vi "XML Script - Set Description of Existing Wire.vi"(9 "Description to Set":string, 10 "Wire Source":string, 11 "Code to Search":string) -> (2 "Wire found?":bool, 3 "Updated Code":string)   [LabVIEW 2017]
uses:
  <vilib>/_script/XML Scripting/XML Script Tag.ctl
  <vilib>/_script/XML Scripting/XML Script Attribute.ctl
panel:
  # "Set description on the first wire in \"Code to Search\"\nwhose source is Wire Source."
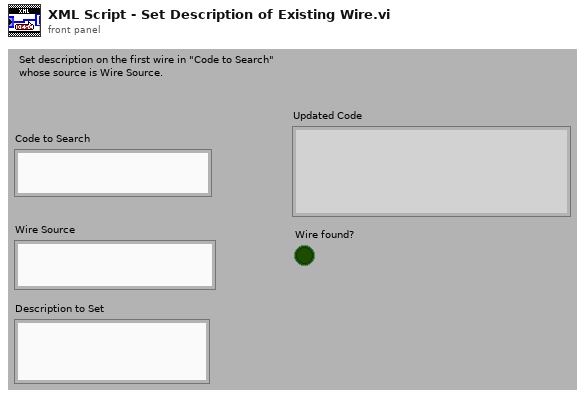
[diagram p1: front panel]
types:
  T1 = typedef "XML Script Attribute.ctl" = enum16{"name", "style", "path", "position", "in", "out", "width", "height", "index", "value", "default", "location", "offset", "typeindex", "size", "source", "destination", "indicator", "type", "controlname", "label", "conpaneidx", "mode", "description", "hasCondTerm", "linkIdentity", "caseselectortype", "concatInputs", "inName", "instantiationpath", "loopCondition", "IndexMode", "formulaInputs", "formulaOutputs", "msnFuncName", "msnIsDynamic", "msnIsODEUserFunction", "ignoreSearchDialog"}
  T2 = typedef "XML Script Tag.ctl" = enum16{"Script", "Function", "SubVI", "GrowableFunction", "Structure", "MultiframeStructure", "Frame", "Tunnel", "ShiftRegister", "Constant", "Control", "Terminal", "Wire", "StaticVIReference", "ControlTerminal", "CompoundArithmetic", "FlatSequence", "FlatSequenceFrame", "MathScriptCallByRef", "BuildArray", "GenericSubVI", "MathScriptNode"}
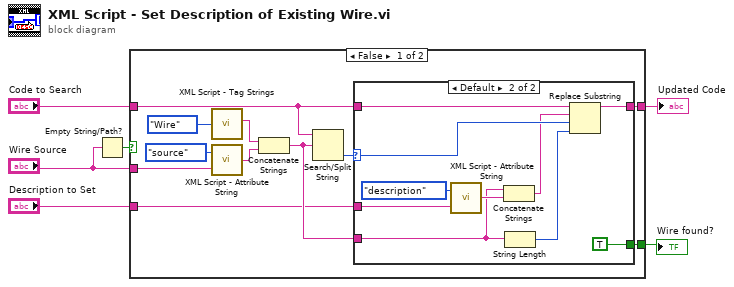
[diagram p0: block diagram]
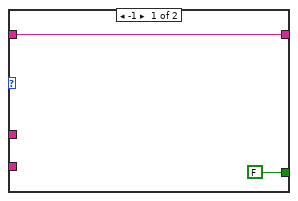
[diagram p2: hidden frame]
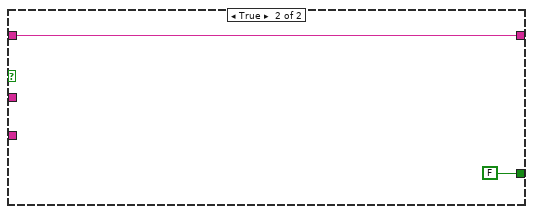
[diagram p3: hidden frame]
diagram:
  n1 = Empty String/Path?(string/path="Wire Source") -> (empty?=w1:bool)
  n2 = case shown="False" w1 {
    tunnel: "Code to Search" -> [w12 w31]
    tunnel: [w11 FALSE ("Wire found?")] -> w5
    tunnel: [w10 w31] -> w4
    tunnel: "Wire Source" -> [w8 _]
    tunnel: "Description to Set" -> [w7 _]
    frame False {
      n3 = call <vilib>:"XML Script - Tag Strings.vi"("XML Script Tag"=XML_Script_Tag."Wire") -> ("XML String - Begin Tag"=w16:string)  [unwired: 2 in, 1 out]
      n4 = call <vilib>:"XML Script - Attribute String.vi"("Attribute String"=w8, "XML Script Attribute"=XML_Script_Attribute."source") -> ("XML Script - Attribute String"=w17:string)
      n5 = Concatenate Strings(w16, w17) -> (w9:string)
      n6 = Search/Split String(string=w12, search string/char (-)=w9) -> (offset of match=w13:i32)  [unwired: 1 in, 2 out]
      n7 = case shown="Default" w13 {
        selector: w13 -> [_ w29]
        tunnel: w7 -> [_ w22]
        tunnel: w12 -> [w18 w21]
        tunnel: [FALSE ("Wire found?") TRUE ("Wire found?")] -> w11
        tunnel: [w18 w23] -> w10
        tunnel: w9 -> [_ w20]
        frame -1 {
        }
        frame Default {
          n8 = call <vilib>:"XML Script - Attribute String.vi"("Attribute String"=w22, "XML Script Attribute"=XML_Script_Attribute."description") -> ("XML Script - Attribute String"=w26:string)
          n9 = Concatenate Strings(w20, w26) -> (w27:string)
          n10 = String Length(string=w20) -> (length=w25:i32)
          n11 = Replace Substring(2:w25, 3:w29, 4:w27, 5:w21) -> (1:w23:string)  [unwired: 1 out]
        }
      }
    }
    frame True {
    }
  }
  "Updated Code" <- w4
  "Wire found?" <- w5
